vi "Write Failure Action Change Event.vi"(10 "Failure Action Change Event":refnum<user-event>, 11 "Input in":refnum<class "Input.lvclass">) -> (3 "Input out":refnum<class "Input.lvclass">)   [LabVIEW 2016, in "AssertEngine.lvlib" / "Input.lvclass"]
uses:
  Input.lvclass
  Input.lvclass/Input.ctl
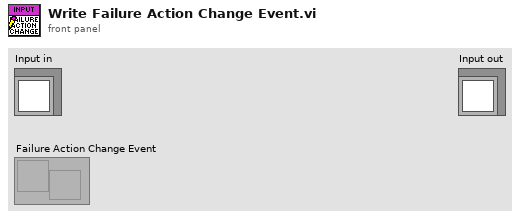
[diagram p1: front panel]
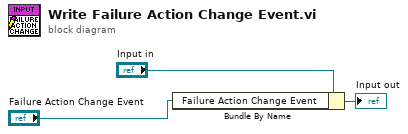
[diagram p0: block diagram]
diagram:
  n1 = Bundle By Name(cluster="Input in", "Failure Action Change Event"="Failure Action Change Event") -> (→"Input out":refnum<class "Input.lvclass">)
